vi "Get Connection List from Indices.vi"(8 "error in (no error)":errorcluster, 10 "Available Relays":i32[](array[numeric]), 11 "SLSC Switch in":refnum<class "SLSC Switch.lvclass">) -> (0 "error out":errorcluster, 2 "String":string, 3 "SLSC Switch out":refnum<class "SLSC Switch.lvclass">)   [LabVIEW 2015, in "SLSC Switch.lvclass"]
uses:
  SLSC Switch.lvclass
  SLSC Switch.lvclass/SLSC Switch.ctl
  Relay Interface/RelayInterface.lvclass
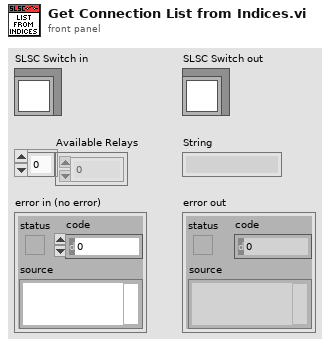
[diagram p1: front panel]
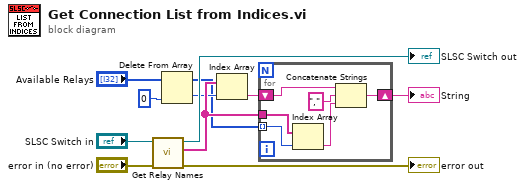
[diagram p0: block diagram]
diagram:
  n1 = call "Get Relay Names.vi"("error in (no error)"="error in (no error)", "SLSC Switch in"="SLSC Switch in") -> ("error out"=→"error out":errorcluster, "Relay Names"=w11:string[], "SLSC Switch out"=→"SLSC Switch out":refnum<class "SLSC Switch.lvclass">)  [unwired: 7 in]
  n2 = Delete From Array(array="Available Relays", index=0) -> (deleted portion=w7:i32, array with subset deleted=w5:i32[])  [unwired: 1 in]
  n3 = Index Array(array=w11, index=w7) -> (element=w8:string)
  n4 = for {
    tunnel: w11 -> [w17]
    tunnel: w5 -> [w16] mode=indexing
    shift-right: [w12] -> w3
    shift-left: w8 -> [w13]
    n5 = Index Array(array=w17, index=w16) -> (element=w15:string)
    n6 = Concatenate Strings(w13, "," ("string"), w15) -> (w12:string)
  }
  "String" <- w3
